vi "Destroy.vi"(8 "Error In":errorcluster, 11 "Communicator in":refnum<class "Communicator.lvclass">) -> (0 "Error Out":errorcluster, 3 "Communicator out":refnum<class "Communicator.lvclass">)   [LabVIEW 2025, in "Communicator.lvclass"]
uses:
  Communicator.lvclass
  <vilib>/ActorFramework/Stop Msg/Stop Msg.lvclass/Stop Msg.ctl
  <vilib>/ActorFramework/Message Enqueuer/Message Enqueuer.lvclass/Message Enqueuer.ctl
  <vilib>/ActorFramework/Message Enqueuer/Enqueue Critical.vi
  <vilib>/ActorFramework/Stop Msg/Stop Msg.lvclass
  <vilib>/Utility/LVClass/Get LV Class Name.vi
  <vilib>/ActorFramework/tracing/Trace Generation/Generate Trace for Message.vi
  <vilib>/ActorFramework/Message Priority Queue/Priority Enqueue.vi
  Interfaces/IConfigure/IConfigure.lvclass
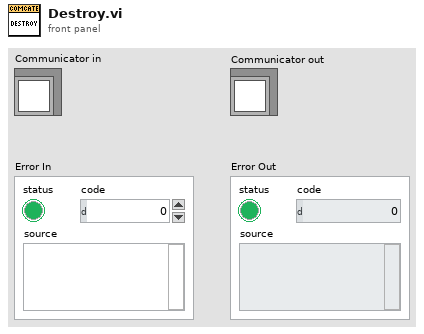
[diagram p1: front panel]
types:
  T1 = typedef "Communicator.lvclass/ObjectAttributes.ctl" = cluster{"IConfigure":refnum<class "IConfigure.lvclass">, "Worker Enqueuer":refnum<class "Message Enqueuer.lvclass">, "Start Counter":i32, "Msg Sent":refnum<user-event>}
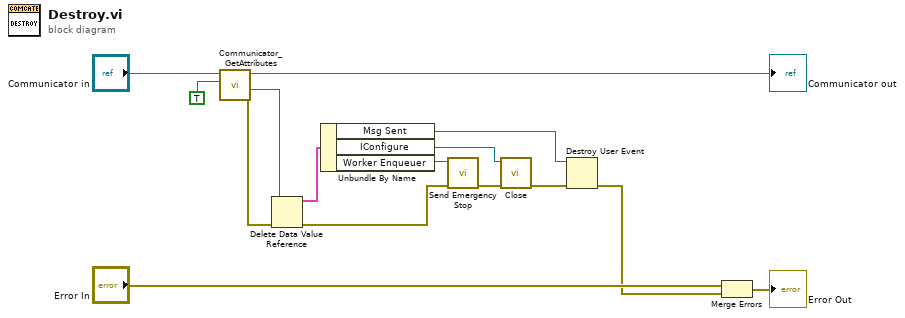
[diagram p0: block diagram]
diagram:
  n1 = call "Communicator_GetAttributes.vi"("OnlyGetDvrReference(False)"=TRUE, "Communicator in"="Communicator in") -> ("Error Out"=w12:errorcluster, "DataRef"=w11:refnum<data-value>, "Communicator out"=→"Communicator out":refnum<class "Communicator.lvclass">)  [unwired: 6 in, 1 out]
  n2 = Delete Data Value Reference(data value reference=w11, error in=w12) -> (data value=w8:T1, error out=w5:errorcluster)
  n3 = Unbundle By Name(w8) -> ("Msg Sent"=w7:refnum<user-event>, "IConfigure"=w1:refnum<class "IConfigure.lvclass">, "Worker Enqueuer"=w4:refnum<class "Message Enqueuer.lvclass">)
  n4 = call <vilib>:"Send Emergency Stop.vi"("error in (no error)"=w5, "Message Enqueuer"=w4) -> ("error out"=w3:errorcluster)  [unwired: 9 in]
  n5 = call-dynamic "Close.vi"("error in"=w3, "IClose in"=w1) -> ("error out"=w2:errorcluster)  [unwired: 8 in, 1 out]
  n6 = Destroy User Event(user event=w7, error in=w2) -> (error out=w6:errorcluster)
  n7 = Merge Errors("Error In", w6) -> (→"Error Out":errorcluster)
